vi "Get States Calling Info.vi"(7 "Data in":T1={"Exit"=FALSE, "States"=enum."Initialize", "Refs"={"Modules"=[], "FGVs"=[]}, "Modules"=[], "Queues Status"=[], "States Calling Info"=[]}, 8 "error in (no error)":errorcluster) -> (0 "error out":errorcluster, 5 "Data out":T1={"Exit"=FALSE, "States"=enum."Initialize", "Refs"={"Modules"=[], "FGVs"=[]}, "Modules"=[], "Queues Status"=[], "States Calling Info"=[]})   [LabVIEW 2019, in "Task Manager.lvlib"]
uses:
  Task Manager.lvlib
  Data.ctl
  Message Queue/State Name.ctl
  Shared/TypeDefs/Queue Info.ctl
  a214c18e-5ce3-44fa-9661-9c13ad52a326.vi
  <vilib>/Utility/error.llb/Clear Errors.vi
  <vilib>/Utility/error.llb/Error Cluster From Error Code.vi
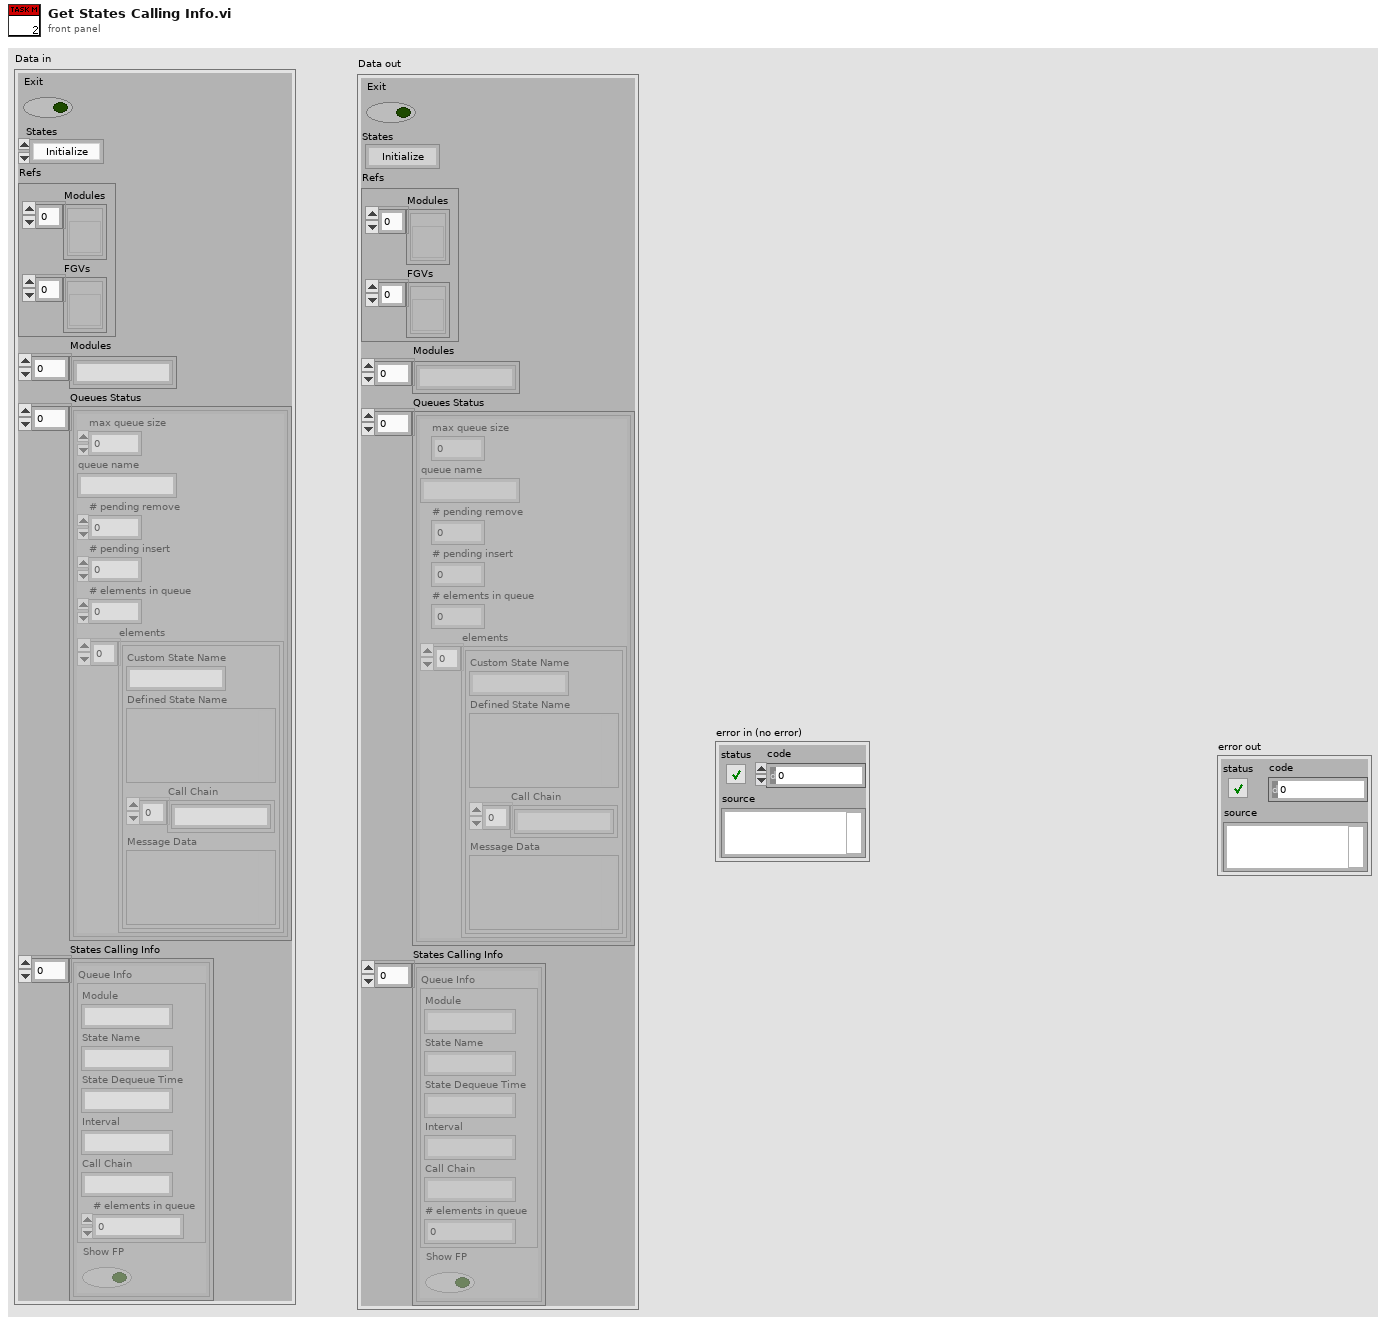
[diagram p1: front panel]
types:
  T1 = typedef "Task Manager.lvlib/Data.ctl" = cluster{"Exit":bool, "States":T2, "Refs":cluster{"Modules":refnum<vi>[], "FGVs":refnum<vi>[]}, "Modules":string[], "Queues Status":cluster{"max queue size":i32, "queue name":string, "# pending remove":i32, "# pending insert":i32, "# elements in queue":i32, "elements":cluster{"Custom State Name":string, "Defined State Name":variant, "Call Chain":string[], "Message Data":variant}[]}[], "States Calling Info":cluster{"Queue Info":T3, "Show FP":bool}[]}
  T2 = typedef "Task Manager.lvlib/State Name.ctl" = enum16{"Default", "Initialize", "Re-Initialize", "Initialize Data", "Initialize Panel", "[Event Structure] Update Data", "Get Modules", "Add State Info Clone", "Get Queue Sizes", "Get States Calling Info", "Error", "Exit"}
  T3 = typedef "Queue Info.ctl" = cluster{"Module":string, "State Name":string, "State Dequeue Time":string, "Interval":string, "Call Chain":string, "# elements in queue":i32}
  T4 = enum32{"Invalid", "Standard", "Closed", "Hidden", "Minimized", "Maximized"}
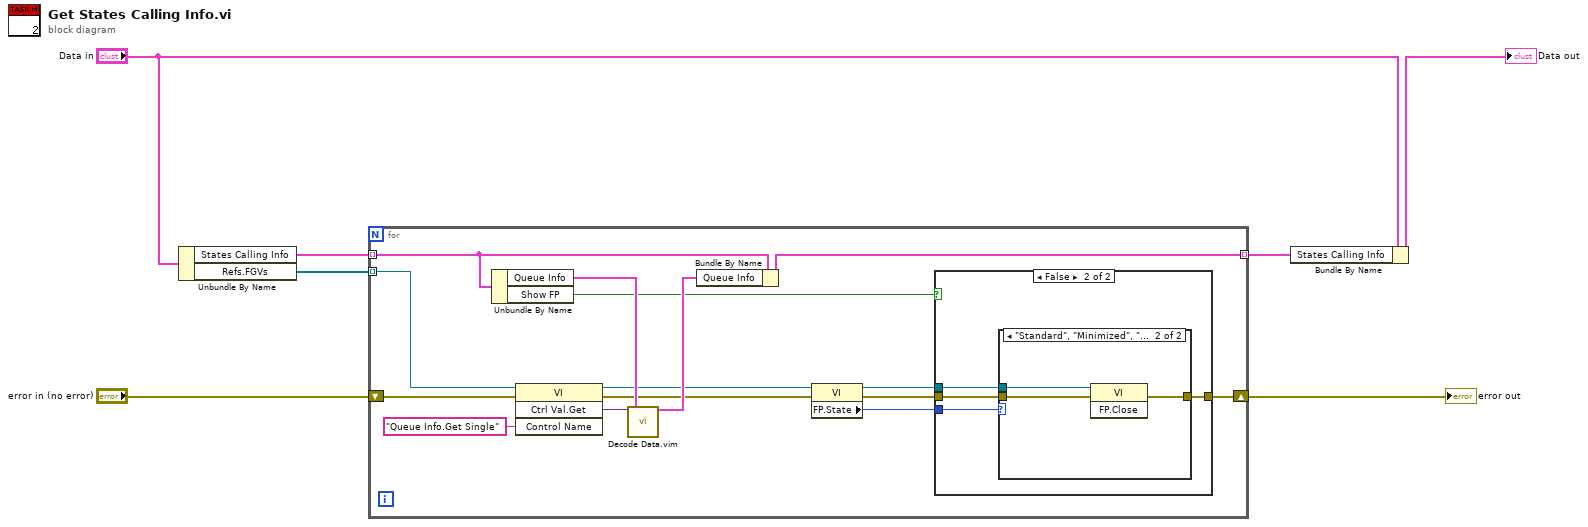
[diagram p0: block diagram]
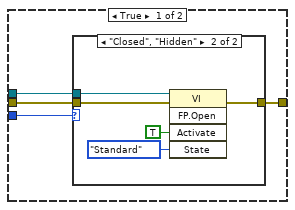
[diagram p2: hidden frame]
diagram:
  n1 = Unbundle By Name("Data in") -> ("States Calling Info"=w2:cluster{"Queue Info":T3, "Show FP":bool}[], "Refs.FGVs"=w5:refnum<vi>[])
  n2 = for {
    tunnel: w5 -> [w20] mode=indexing
    tunnel: [w17] -> w1 mode=indexing
    shift-right: [w16] -> w3
    shift-left: "error in (no error)" -> [w19]
    tunnel: w2 -> [w15] mode=indexing
    n3 = Unbundle By Name(w15) -> ("Queue Info"=w14:T3, "Show FP"=w9:bool)
    n4 = invoke class="VI" method="Ctrl Val.Get"(reference=w20, error in=w19, "Control Name"="Queue Info.Get Single") -> (reference out=w12:refnum<vi>, error out=w13:errorcluster, "Get Control Value Variant"=w21:variant)  [unwired: 1 in, 1 out]
    n5 = call "Decode Data.vim"("Data"=w21, "Type/Default value"=w14) -> ("Data out"=w18:T3)  [unwired: 16 in, 1 out]
    n6 = Bundle By Name(cluster=w15, "Queue Info"=w18) -> (w17:cluster{"Queue Info":T3, "Show FP":bool})
    n7 = property class="VI"(reference=w12, error in=w13) -> (reference out=w11:refnum<vi>, error out=w10:errorcluster, "FP.State"=w8:T4)
    n8 = case shown="False" w9 {
      tunnel: w10 -> [w26 w35]
      tunnel: w11 -> [w25 w34]
      tunnel: [w24 w33] -> w16
      tunnel: w8 -> [w23 w32]
      frame True {
        n9 = case shown="\"Closed\", \"Hidden\"" w23 {
          tunnel: w26 -> [w27 w31]
          tunnel: w25 -> [_ w28]
          tunnel: [w27 w31] -> w24
          frame "Invalid", Default {
          }
          frame "Closed", "Hidden" {
            n10 = invoke class="VI" method="FP.Open"(reference=w28, "Activate"=TRUE ("Activate?"), "State"=T4."Standard") -> ()  [unwired: 2 in, 5 out]
          }
        }
      }
      frame False {
        n11 = case shown="\"Standard\", \"Minimized\", \"Maximized\"" w32 {
          tunnel: w35 -> [w36 w39]
          tunnel: w34 -> [_ w38]
          tunnel: [w36 w37] -> w33
          frame "Invalid", Default {
          }
          frame "Standard", "Minimized", "Maximized" {
            n12 = invoke class="VI" method="FP.Close"(reference=w38, error in=w39) -> (error out=w37:errorcluster)  [unwired: 1 in, 2 out]
          }
        }
      }
    }
  }
  "error out" <- w3
  n13 = Bundle By Name(cluster="Data in", "States Calling Info"=w1) -> (→"Data out":T1)
